vi "OEE_PART_1.vi"(8 "Number of days":dbl, 9 "CYCLE TIME":string[](array[string]), 10 "ACTUAL PROD TIME":string[](array[string]), 11 "BREAKDOWN TOTAL TIME":string[][](array[string])) -> (0 "Availability Time":dbl, 1 "Numeric":i32, 2 "CAPACITY":dbl, 3 "ACTUAL TIME":i32)   [LabVIEW 2017]
panel:
  out "subarray":string[](array[string])
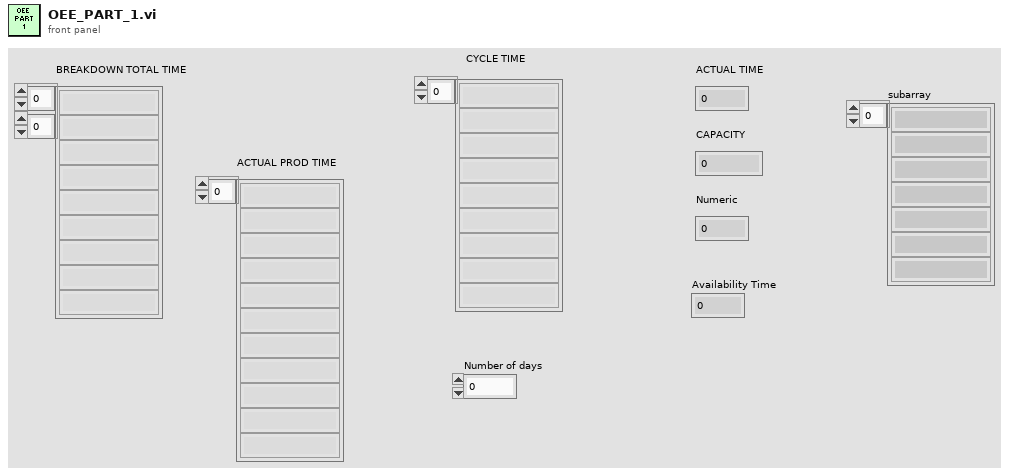
[diagram p1: front panel]
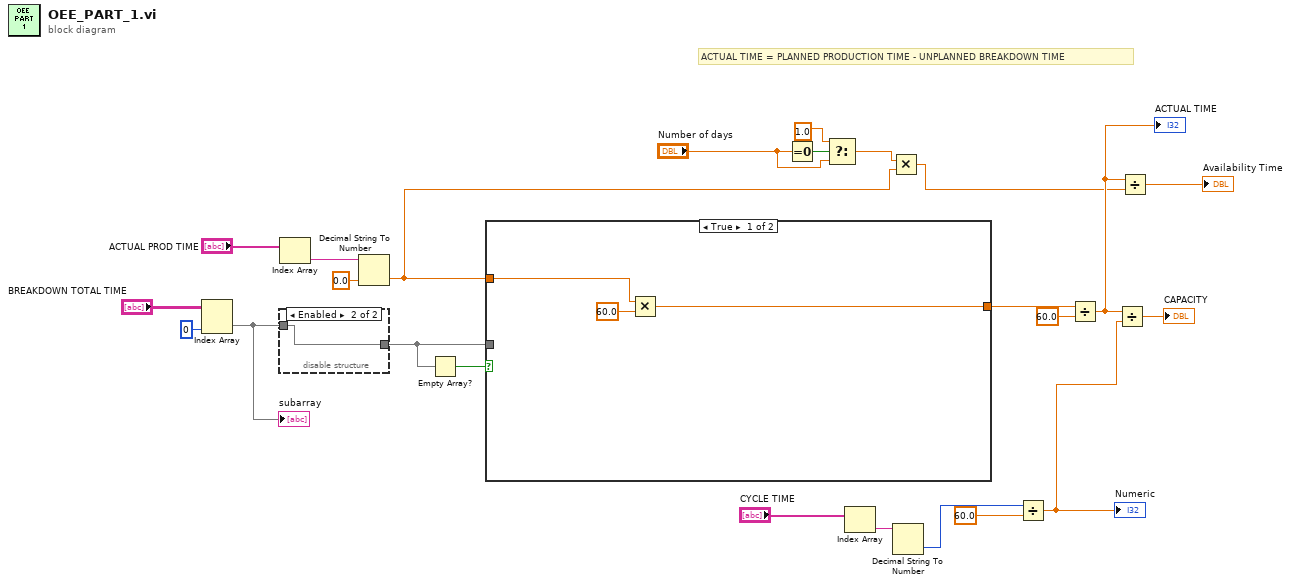
[diagram p0: block diagram]
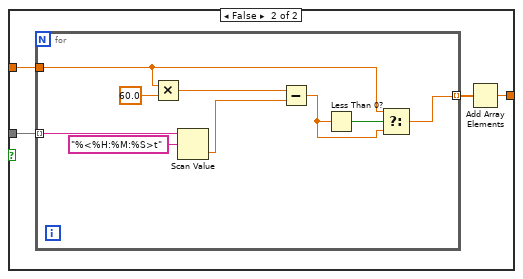
[diagram p2: hidden frame]
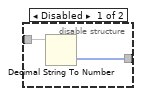
[diagram p3: hidden frame]
diagram:
  # "ACTUAL TIME = PLANNED PRODUCTION TIME - UNPLANNED BREAKDOWN TIME"
  n1 = Index Array(array="BREAKDOWN TOTAL TIME", index (col)=0 ("disabled index (col)")) -> (element=w16:string[])  [unwired: 1 in]
  "subarray" <- w16
  n2 = Index Array(array="ACTUAL PROD TIME") -> (element=w21:string)  [unwired: 1 in]
  n3 = disable-structure shown="Enabled" {
    disable-tunnel: w16 -> [w26 w27]
    disable-tunnel: [w25 w27] -> w3
    frame Disabled {
      n4 = Decimal String To Number(string=w26) -> (number=w25:i32[])  [unwired: 2 in, 1 out]
    }
    frame Enabled {
    }
  }
  n5 = Decimal String To Number(string=w21, default (0L)=0.0 ("default (0 I32)")) -> (number=w5:dbl)  [unwired: 1 in, 1 out]
  n6 = Empty Array?(array=w3) -> (empty?=w2:bool)
  n7 = case shown="True" w2 {
    tunnel: w5 -> [w30 w34]
    tunnel: w3 -> [_ w33]
    tunnel: [w28 w32] -> w1
    frame True {
      n8 = Multiply(x=w30, y=60.0) -> (x*y=w28:dbl)
    }
    frame False {
      n9 = for {
        tunnel: w34 -> [w36]
        tunnel: [w35] -> w31 mode=indexing
        tunnel: w33 -> [w42] mode=indexing
        n10 = Multiply(x=w36, y=60.0) -> (x*y=w40:dbl)
        n11 = Scan Value(string=w42, format string="%<%H:%M:%S>t") -> (value=w39:dbl)  [unwired: 1 in, 1 out]
        n12 = Subtract(x=w40, y=w39) -> (x-y=w37:dbl)
        n13 = Less Than 0?(x=w37) -> (x < 0?=w38:bool)
        n14 = Select(t=w36, s=w38, f=w37) -> (s? t:f=w35:dbl)
      }
      n15 = Add Array Elements(numeric array=w31) -> (sum=w32:dbl)
    }
  }
  n16 = Equal To 0?(x="Number of days") -> (x = 0?=w9:bool)
  n17 = Select(t=1.0, s=w9, f="Number of days") -> (s? t:f=w6:dbl)
  n18 = Index Array(array="CYCLE TIME") -> (element=w23:string)  [unwired: 1 in]
  n19 = Multiply(x=w6, y=w5) -> (x*y=w4:dbl)
  n20 = Decimal String To Number(string=w23) -> (number=w13:i32)  [unwired: 2 in, 1 out]
  n21 = Divide(x=w13, y=60.0) -> (x/y=w12:dbl)
  "Numeric" <- w12
  n22 = Divide(x=w1, y=60.0) -> (x/y=w11:dbl)
  "ACTUAL TIME" <- w11
  n23 = Divide(x=w11, y=w12) -> (x/y=→"CAPACITY":dbl)
  n24 = Divide(x=w11, y=w4) -> (x/y=→"Availability Time":dbl)
